vi "Create DSF Configuration Session v2.vi"(8 "error in (no error)":errorcluster, 10 "config data":T1) -> (0 "error out":errorcluster, 3 "DSF Configuration Session out":T15)   [LabVIEW 2017, in "DSF Configuration.lvlib" / "Configuration Session.lvclass"]
uses:
  Configuration Session.lvclass
  DSF Configuration API/Private/Controls/Session/DSF Configuration Reference.ctl
  DSF Configuration API/Private/Controls/DSF File Format/Internal.DSF Configuration.ctl
  DSF Configuration API/Public/Controls/DSF Version Info.ctl
  DSF Configuration API/Private/Controls/DSF File Format/Internal.DSF Plugin with ID.ctl
  DSF Configuration API/Private/Controls/DSF File Format/Internal.DSF Plugin Info.ctl
  DSF Configuration API/Public/Controls/DSF Timing Info.ctl
  DSF Configuration API/Private/Controls/DSF File Format/Internal.DSF Group with ID.ctl
  DSF Configuration API/Private/Controls/DSF File Format/Internal.DSF Group Info.ctl
  DSF Configuration API/Private/Controls/DSF File Format/Internal.DSF Transfer with ID.ctl
  DSF Configuration API/Private/Controls/DSF File Format/Internal.DSF Transfer Info.ctl
  DSF Configuration API/Private/Controls/DSF File Format/Internal.DSF Channel with ID.ctl
  DSF Configuration API/Private/Controls/DSF File Format/Internal.DSF Channel Info.ctl
  DSF Configuration API/Private/Controls/DSF File Format/Internal.DSF Settings with ID.ctl
  DSF Configuration API/Private/Controls/DSF File Format/Internal.DSF Settings Info.ctl
  DSF Configuration API/Private/Controls/Session/DSF Config Data.ctl
  DSF Configuration.lvlib
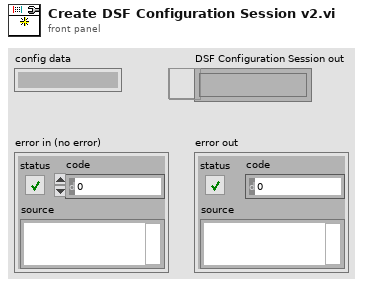
[diagram p1: front panel]
types:
  T1 = typedef "DSF Configuration.lvlib/Configuration Session.lvclass/DSF Config Data.ctl" = cluster{"dsf configuration":T2, "path":path, "dirty":bool}
  T2 = typedef "DSF Configuration.lvlib/Configuration Session.lvclass/Internal.DSF Configuration.ctl" = cluster{"dsfversion":T3, "version":T3, "plugins":T4[], "groups":T7[], "transfers":T9[], "channels":T11[], "settings":T13[]}
  T3 = typedef "DSF Configuration.lvlib/DSF Version Info.ctl" = cluster{"major":u32, "minor":u32, "fix":u32, "build":string}
  T4 = typedef "DSF Configuration.lvlib/Configuration Session.lvclass/Internal.DSF Plugin with ID.ctl" = cluster{"id":string, "values":T5}
  T5 = typedef "DSF Configuration.lvlib/Configuration Session.lvclass/Internal.DSF Plugin Info.ctl" = cluster{"type":string, "timing":T6, "group ids":string[], "settings id":string}
  T6 = typedef "DSF Configuration.lvlib/DSF Timing Info.ctl" = cluster{"priority":u64, "decimation":u64, "offset":u64}
  T7 = typedef "DSF Configuration.lvlib/Configuration Session.lvclass/Internal.DSF Group with ID.ctl" = cluster{"id":string, "values":T8}
  T8 = typedef "DSF Configuration.lvlib/Configuration Session.lvclass/Internal.DSF Group Info.ctl" = cluster{"direction":i32, "timing":T6, "transfer ids":string[], "settings id":string}
  T9 = typedef "DSF Configuration.lvlib/Configuration Session.lvclass/Internal.DSF Transfer with ID.ctl" = cluster{"id":string, "values":T10}
  T10 = typedef "DSF Configuration.lvlib/Configuration Session.lvclass/Internal.DSF Transfer Info.ctl" = cluster{"byte order":i32, "channel ids":string[], "settings id":string}
  T11 = typedef "DSF Configuration.lvlib/Configuration Session.lvclass/Internal.DSF Channel with ID.ctl" = cluster{"id":string, "values":T12}
  T12 = typedef "DSF Configuration.lvlib/Configuration Session.lvclass/Internal.DSF Channel Info.ctl" = cluster{"count":u64, "buffer offset":u64, "data type":i32, "settings id":string}
  T13 = typedef "DSF Configuration.lvlib/Configuration Session.lvclass/Internal.DSF Settings with ID.ctl" = cluster{"id":string, "values":T14}
  T14 = typedef "DSF Configuration.lvlib/Configuration Session.lvclass/Internal.DSF Settings Info.ctl" = cluster{"key":string, "value":string}[]
  T15 = typedef "DSF Configuration.lvlib/Configuration Session.lvclass/DSF Configuration Reference.ctl" = refnum<data-value>
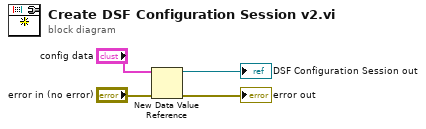
[diagram p0: block diagram]
diagram:
  n1 = New Data Value Reference(data value="config data", error in="error in (no error)") -> (data value reference=→"DSF Configuration Session out":refnum<data-value>, error out=→"error out":errorcluster)
